vi "Celda solar.vi"() -> ()   [LabVIEW 2014]
uses:
  <vilib>/imath/engines/lvmath2/RunTimeEngine/ArithmeticOperatorToken/NIMS_ArithmeticOperator_power(S).vi
  <instcachedir>/0/NIMS_ArithmeticOperator_power(S)_CAFE680B12A64A3A8F5E28A20C679B7D.lvgen/NIMS_ArithmeticOperator_power(S)_CAFE680B12A64A3A8F5E28A20C679B7D_014.vi
  <vilib>/imathl/engines/lvmath/Functions/Error Handling/Create Error.vi
  <vilib>/imath/engines/lvmath2/RunTimeEngine/CommandStatement/MC_CommandStatement_break.vi
  <vilib>/imath/engines/lvmath2/RunTimeEngine/RangeToken/NIMS_Range_R2 - Integer.vi
  <instcachedir>/0/NIMS_Range_R2 - Integer_2D1304BAF97744E0A293025746CBADFC.lvgen/NIMS_Range_R2 - Integer_2D1304BAF97744E0A293025746CBADFC_000.vi
  <vilib>/imath/engines/lvmath2/RunTimeEngine/IndexReplace/NIMS V(S)=S.vi
  <instcachedir>/0/NIMS V(S)=S_2D52C4EC15D8415E870AEE69FB516CCA.lvgen/NIMS V(S)=S_2D52C4EC15D8415E870AEE69FB516CCA_001.vi
  <instcachedir>/0/NIMS V(S)=S_2D52C4EC15D8415E870AEE69FB516CCA.lvgen/NIMS V(S)=S_2D52C4EC15D8415E870AEE69FB516CCA_000.vi
  <vilib>/imath/engines/lvmath2/RunTimeEngine/CommandStatement/NIMS_CommandStatement_MaskErr.vi
  <vilib>/imath/engines/lvmath2/RunTimeEngine/NodeEndStatement/NIMS_NodeEndStatement_Output.vi
  <instcachedir>/0/NIMS_NodeEndStatement_Output_53EC0D466D134D7ABD903AC30B43404B.lvgen/NIMS_NodeEndStatement_Output_53EC0D466D134D7ABD903AC30B43404B_000.vi
  <instcachedir>/0/NIMS_NodeEndStatement_Output_53EC0D466D134D7ABD903AC30B43404B.lvgen/NIMS_NodeEndStatement_Output_53EC0D466D134D7ABD903AC30B43404B_005.vi
  <vilib>/imath/engines/lvmath2/RunTimeEngine/ErrorHandling/NIMS_Finalize Error.vi
panel:
  in  "Eliminar curvas":bool
  in  "Almacenar imagen":bool
  in  "Array":cluster{i32[], "sine wave":dbl[]}[](array[cluster])
  in  "Trazar curva":bool
  out "Curva Caracteristica I-V":cluster{"Vao":dbl[], "Iao":dbl[]}[](graph)
  out "Ia":cdb[](array[numeric])
  in  "Celdas en serie":dbl
  in  "Irradiación":dbl caption="Radiaccion" step=0.05
  in  "Temperatura":dbl
  in  "stop":bool
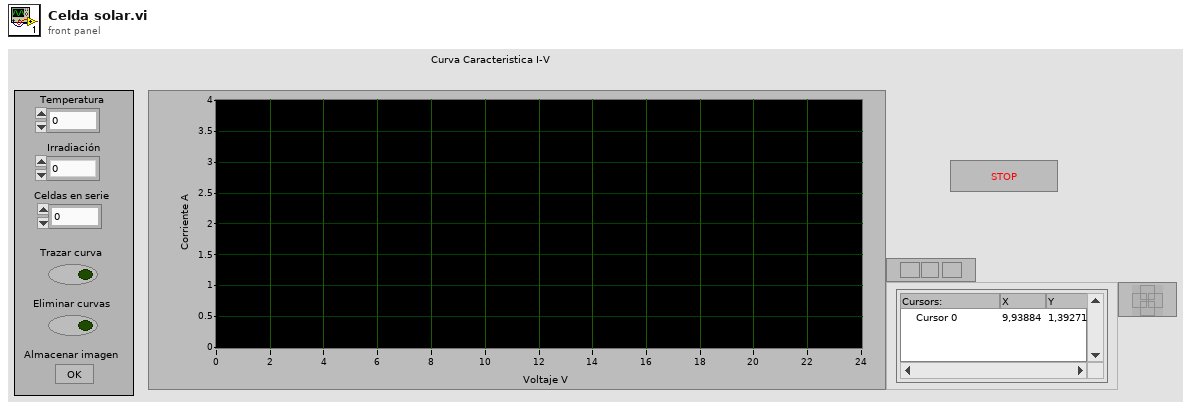
[diagram p1: front panel]
types:
  T1 = typedef "imagedata.ctl" = cluster{"image type":i32, "image depth":i32, "image":u8[], "mask":u8[], "colors":u32[], "Rectangle":cluster{"left":i16, "top":i16, "right":i16, "bottom":i16}}
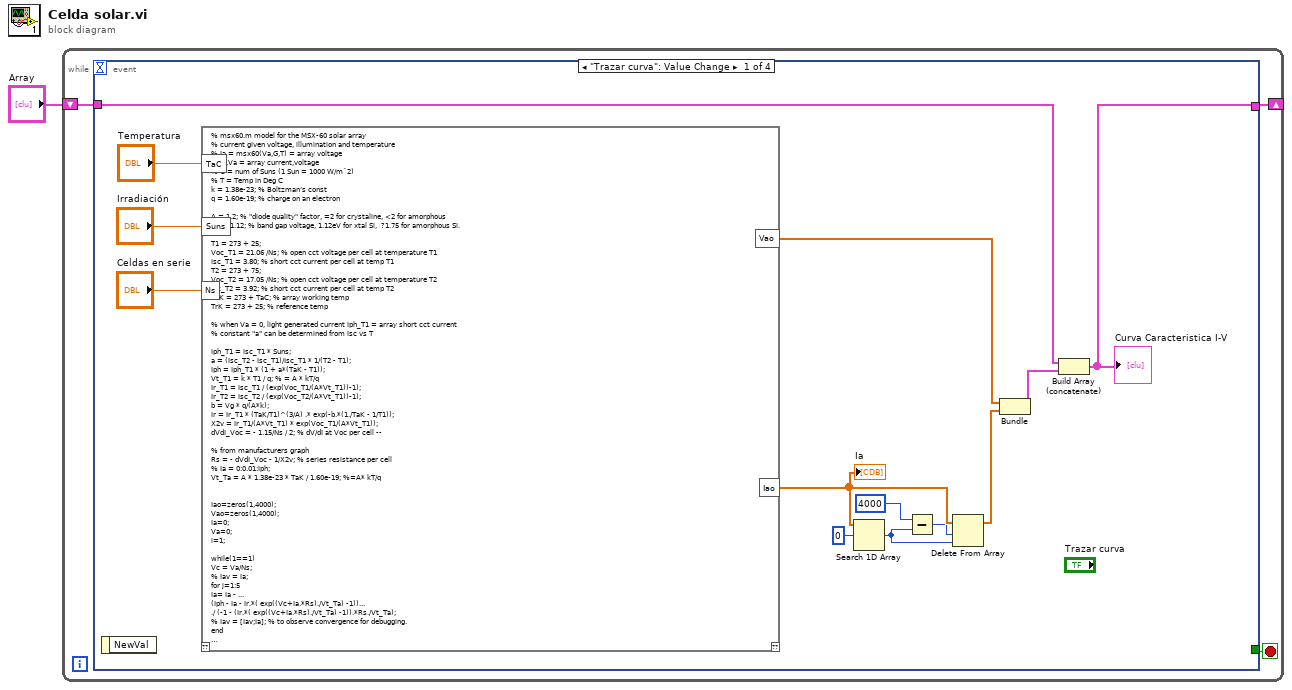
[diagram p0: block diagram]
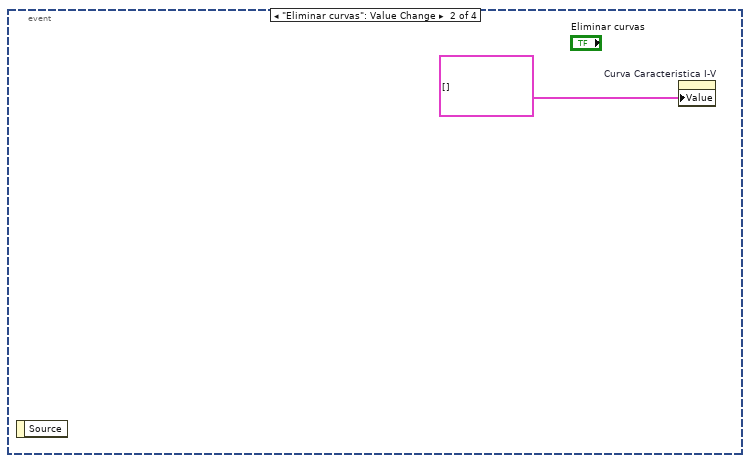
[diagram p2: hidden frame]
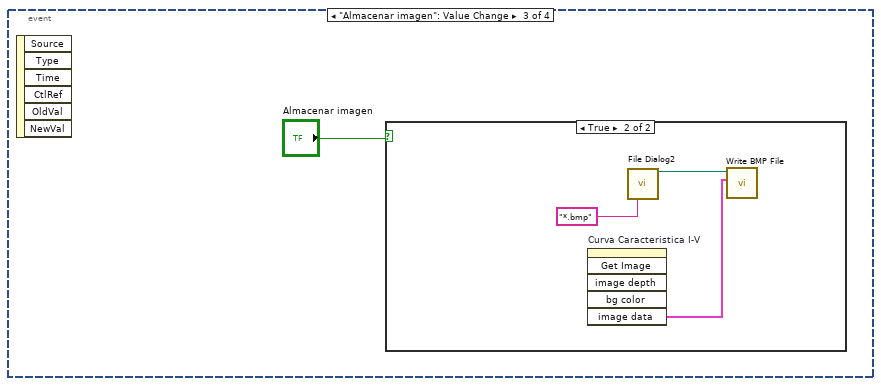
[diagram p3: hidden frame]
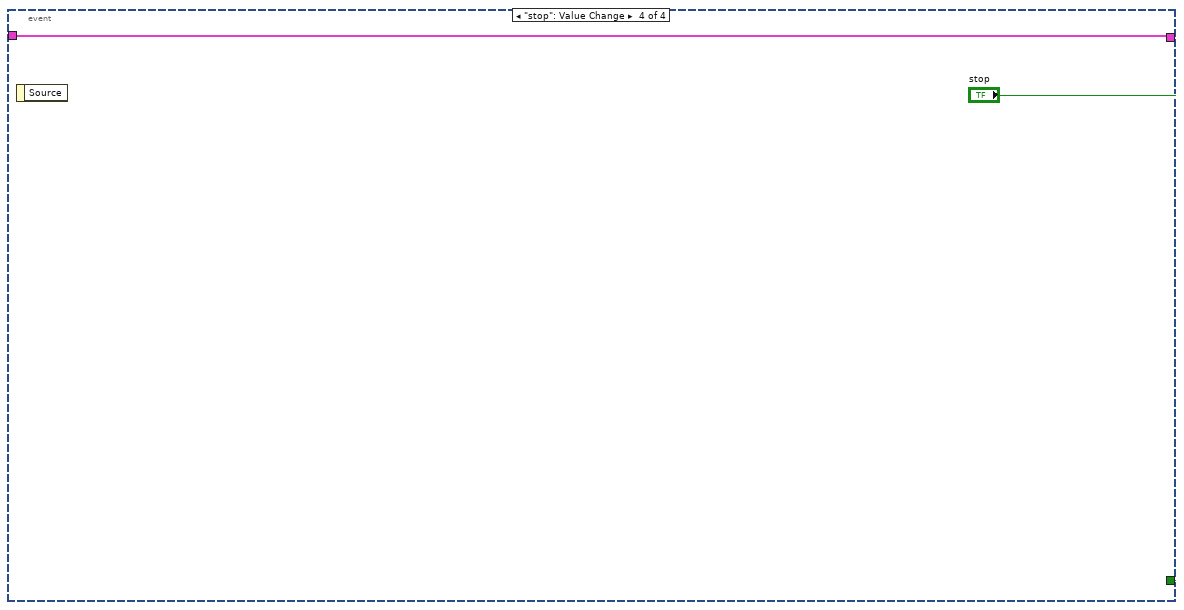
[diagram p5: hidden frame]
diagram:
  n1 = while {
    shift-right: [w3] -> _
    shift-left: "Array" -> [w4]
    stop <- w2 stop-if-true
    n2 = event shown="[0] \"Trazar curva\": Value Change" {
      selector: _ -> [_ _ _ _]
      dyn-events: _ -> [_ _ _ _]
      timeout: _ -> [_ _ _ _]
      tunnel: w4 -> [w6 _ _ w547]
      tunnel: [w5 _ _ w547] -> w3
      tunnel: [_ _ _ "stop"] -> w2
      event "Trazar curva": Value Change {
        n3 = event-data() -> ()  [unwired: 1 in, 1 out]
        n4 = mathscript code="% msx60.m model for the MSX-60 solar array\n% current given voltage, illumination and temperature\n% Ia = msx60(Va,G,T) = array voltage\n% Ia,Va = array current,voltage\n% G = num of Suns (1 Sun = 1000 W/mˆ2)\n% T = Temp in Deg C\nk = 1.38e-23; % Boltzman’s const\nq = 1.60e-19; % charge on an electron\n\nA = 1.2; % \"diode quality\" factor, =2 for crystaline, <2 for amorphous\nVg = 1.12; % band gap voltage, 1.12eV for xtal Si,  ?1.75 for amorphous Si.\n\nT1 = 273 + 25;\nVoc_T1 = 21.06 /Ns; % open cct voltage per cell at temperature T1\nIsc_T1 = 3.80; % short cct current per cell at temp T1\nT2 = 273 + 75;\nVoc_T2 = 17.05 /Ns; % open cct voltage per cell at temperature T2\nIsc_T2 = 3.92; % short cct current per cell at temp T2\nTaK = 273 + TaC; % array working temp\nTrK = 273 + 25; % reference temp\n\n% when Va = 0, light generated current Iph_T1 = array short cct current\n% constant \"a\" can be determined from Isc vs T\n\nIph_T1 = Isc_T1 * Suns;\na = (Isc_T2 - Isc_T1)/Isc_T1 * 1/(T2 - T1);\nIph = Iph_T1 * (1 + a*(TaK - T1));\nVt_T1 = k * T1 / q; % = A * kT/q\nIr_T1 = Isc_T1 / (exp(Voc_T1/(A*Vt_T1))-1);\nIr_T2 = Isc_T2 / (exp(Voc_T2/(A*Vt_T1))-1);\nb = Vg * q/(A*k);\nIr = Ir_T1 * (TaK/T1)^(3/A) .* exp(-b.*(1./TaK - 1/T1));\nX2v = Ir_T1/(A*Vt_T1) * exp(Voc_T1/(A*Vt_T1));\ndVdI_Voc = - 1.15/Ns / 2; % dV/dI at Voc per cell --\n\n% from manufacturers graph\nRs = - dVdI_Voc - 1/X2v; % series resistance per cell\n% Ia = 0:0.01:Iph;\nVt_Ta = A * 1.38e-23 * TaK / 1.60e-19; %=A* kT/q\n\n\nIao=zeros(1,4000);\nVao=zeros(1,4000);\nIa=0;\nVa=0;\ni=1;\n\nwhile(1==1)\nVc = Va/Ns;\n% Iav = Ia;\nfor j=1:5\nIa= Ia - ...\n(Iph - Ia - Ir.*( exp((Vc+Ia.*Rs)./Vt_Ta) -1))...\n./ (-1 - (Ir.*( exp((Vc+Ia.*Rs)./Vt_Ta) -1)).*Rs./Vt_Ta);\n% Iav = [Iav;Ia]; % to observe convergence for debugging.\nend\n\nif(Ia<=0) break\nend\n\nIao(i)=Ia;\nVao(i)=Va;\n\ni=i+1;\nVa=Va+1/100;\n\nend"("TaC"="Temperatura", "Suns"="Irradiación", "Ns"="Celdas en serie") -> ("Iao"=w16:cdb[], "Vao"=w17:dbl[])  [unwired: 1 in, 1 out]
        "Ia" <- w16
        n5 = Search 1D Array(1D array=w16, element=0) -> (index of element=w9:i32)  [unwired: 1 in]
        n6 = Subtract(x=4000, y=w9) -> (x-y=w10:i32)
        n7 = Delete From Array(array=w16, length=w10, index=w9) -> (array with subset deleted=w8:cdb[])  [unwired: 1 out]
        n8 = Bundle("Vao"=w17, "Iao"=w8) -> (w7:cluster{"Vao":dbl[], "Iao":cdb[]})  [unwired: 1 in]
        n9 = Build Array (concatenate)(w6, w7) -> (w5:cluster{"Vao":dbl[], "Iao":cdb[]}[])
        "Curva Caracteristica I-V" <- w5
      }
      event "Eliminar curvas": Value Change {
        n10 = event-data() -> ()  [unwired: 1 in, 1 out]
        n11 = property on="Curva Caracteristica I-V" class="XYGraph (strict)"("Value"=cluster{"Vao":dbl[], "Iao":dbl[]}[] [] ("Curva Caracteristica I-V")) -> ()  [unwired: 2 in, 2 out]
      }
      event "Almacenar imagen": Value Change {
        n12 = event-data() -> ()  [unwired: 1 in, 6 out]
        n13 = case shown="True" "Almacenar imagen" {
          frame False {
          }
          frame True {
            n14 = invoke on="Curva Caracteristica I-V" class="XYGraph (strict)" method="Get Image"() -> ("image data"=w545:T1)  [unwired: 6 in, 5 out]
            n15 = call "File Dialog2"("pattern (all files)"="*.bmp") -> ("selected path"=w544:path)  [unwired: 11 in, 3 out]
            n16 = call <vilib>:"Write BMP File.vi"("image data"=w545, "path to BMP file"=w544) -> ()  [unwired: 8 in, 2 out]
          }
        }
      }
      event "stop": Value Change {
        n17 = event-data() -> ()  [unwired: 1 in, 1 out]
      }
    }
  }
